vi "Find First Matching Resource (U32).vi"(6 "Error if not found? (F)":bool, 8 "Error in":errorcluster caption="Error in (no error)", 10 "Resource Types":u32[](array[numeric]), 11 "Resources":T1) -> (0 "Error out":errorcluster, 1 "Index":i32, 2 "Found?":bool, 3 "Resource":T2)   [LabVIEW 2018, in "Resource Manipulation.lvlib"]
uses:
  Resource Manipulation.lvlib
  Resource.ctl
  Resource Array.ctl
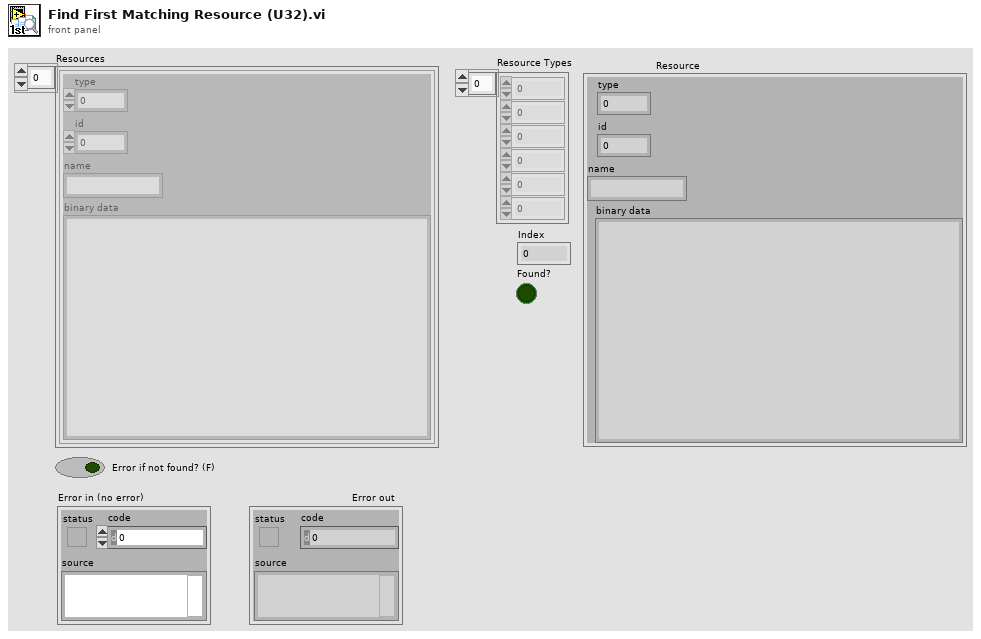
[diagram p1: front panel]
types:
  T1 = typedef "Resource Manipulation.lvlib/Resource Array.ctl" = T2[]
  T2 = typedef "Resource Manipulation.lvlib/Resource.ctl" = cluster{"type":u32, "id":i32, "name":string, "binary data":string}
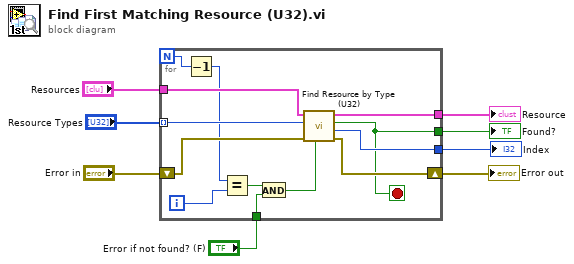
[diagram p0: block diagram]
diagram:
  n1 = for {
    N -> [w11]
    tunnel: "Resource Types" -> [w21] mode=indexing
    tunnel: "Resources" -> [w20]
    shift-right: [w17] -> w5
    shift-left: "Error in" -> [w18]
    tunnel: [w19] -> w7
    tunnel: "Error if not found? (F)" -> [w13]
    tunnel: [w10] -> w2
    tunnel: [w9] -> w1
    i -> [w15]
    stop <- w9 stop-if-true
    n2 = Decrement(x=w11) -> (x-1=w16:i32)
    n3 = Equal?(x=w16, y=w15) -> (x = y?=w14:bool)
    n4 = And(x=w14, y=w13) -> (x .and. y?=w12:bool)
    n5 = call "Find Resource by Type (U32).vi"("Error if not found? (F)"=w12, "Error in"=w18, "Resource Type"=w21, "Resources"=w20) -> ("Error out"=w17:errorcluster, "Index"=w10:i32, "Found?"=w9:bool, "Resource"=w19:T2)  [unwired: 4 in]
  }
  "Error out" <- w5
  "Index" <- w2
  "Resource" <- w7
  "Found?" <- w1
